vi "Scale mm To um.vi"() -> ()   [LabVIEW 2015, in "Utility.lvlib"]
uses:
  Utility.lvlib
panel:
  out "um":dbl
  in  "mm":dbl
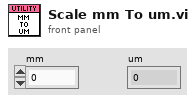
[diagram p1: front panel]
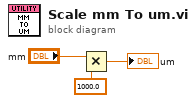
[diagram p0: block diagram]
diagram:
  n1 = Multiply(x="mm", y=1000.0) -> (x*y=→"um":dbl)
